vi "Do Local Msg Set.vi"(10 "Variant (X Actor.lvclass)":variant) -> (2 "Local Msg Set":T1)   [LabVIEW 2025, in "jettl.lvlib" / "Actor.lvlib"]
uses:
  Actor.lvlib
  Msg Set.ctl
  Msg/Msg.lvclass
  <vilib>/Utility/Data Type/NI_Data Type.lvlib
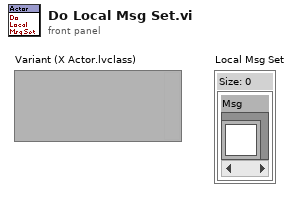
[diagram p1: front panel]
types:
  T1 = typedef "jettl.lvlib/Actor.lvlib/Msg Set.ctl" = set{refnum<class "Msg.lvclass">}
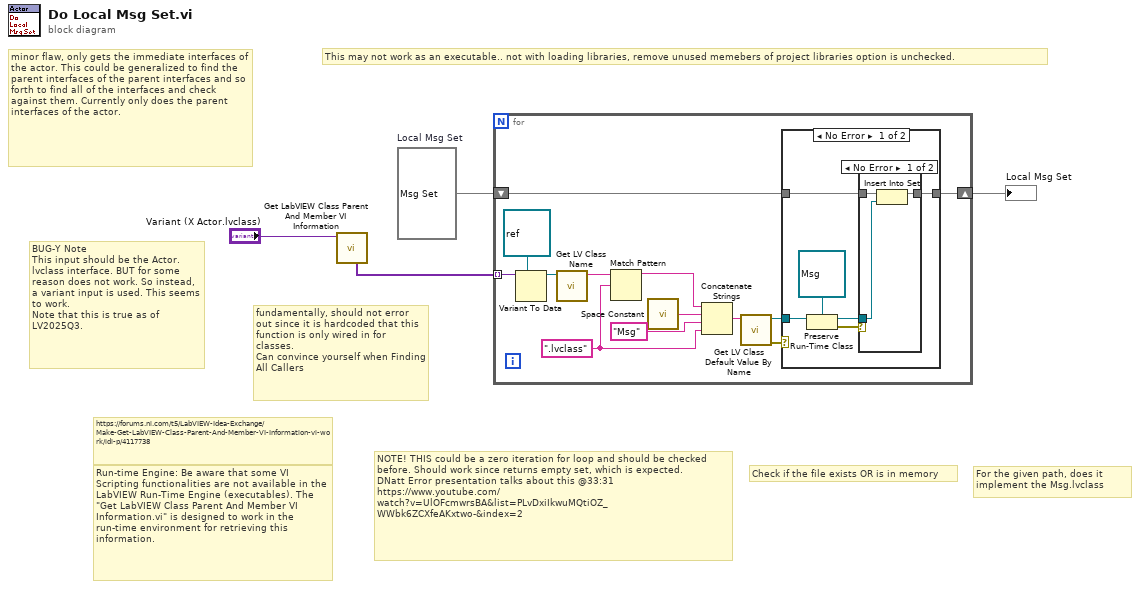
[diagram p0: block diagram]
diagram:
  w1 = T1 {}  # Local Msg Set
  # "fundamentally, should not error out since it is hardcoded that this function is only wired in for classes.\nCan convince yourself when Finding All Callers"
  # "Check if the file exists OR is in memory"
  # "For the given path, does it implement the Msg.lvclass"
  # "NOTE! THIS could be a zero iteration for loop and should be checked before. Should work since returns empty set, which is expected.\nDNatt Error presentation talks about this @33:31\nhttps://www.youtube.com/watch?v=UlOFcmwrsBA&list=PLvDxiIkwuMQtiOZ_WWbk6ZCXfeAKxtwo-&index=2"
  # "BUG-Y Note\nThis input should be the Actor.lvclass interface. BUT for some reason does not work. So instead, a variant input is used. This seems to work.\nNote that this is true as of LV2025Q3."
  # "minor flaw, only gets the immediate interfaces of the actor. This could be generalized to find the parent interfaces of the parent interfaces and so forth to find all of the interfaces and check against them. Currently only does the parent interfaces of the actor."
  # "This may not work as an executable.. not with loading libraries, remove unused memebers of project libraries option is unchecked."
  # "Run-time Engine: Be aware that some VI Scripting functionalities are not available in the LabVIEW Run-Time Engine (executables). The \"Get LabVIEW Class Parent And Member VI Information.vi\" is designed to work in the run-time environment for retrieving this information."
  # "https://forums.ni.com/t5/LabVIEW-Idea-Exchange/Make-Get-LabVIEW-Class-Parent-And-Member-VI-Information-vi-work/idi-p/4117738"
  n1 = call <vilib>:"Get LabVIEW Class Parent And Member VI Information.vi"("variant"="Variant (X Actor.lvclass)") -> ("parent interfaces"=w4:variant[])  [unwired: 7 in, 3 out]
  n2 = for {
    tunnel: w4 -> [w16] mode=indexing
    shift-right: [w12] -> w3
    shift-left: w1 -> [w13]
    w9 = ".lvclass" ("string")
    n3 = Variant To Data(type=refnum<class> refnum ("LabVIEW Object"), Variant=w16) -> (data=w15:refnum<class>)  [unwired: 1 in, 1 out]
    n4 = call <vilib>:"Get LV Class Name.vi"("object"=w15) -> ("class name"=w11:string)  [unwired: 9 in, 1 out]
    n5 = Match Pattern(string=w11, regular expression=w9) -> (before substring=w8:string)  [unwired: 1 in, 3 out]
    n6 = call <vilib>:"Space Constant.vi"() -> ("String"=w7:string)
    n7 = Concatenate Strings(w8, w7, "Msg" ("string"), w9) -> (w6:string)
    n8 = call <vilib>:"Get LV Class Default Value By Name.vi"("class name"=w6) -> ("error out"=w5:errorcluster, "object"=w14:refnum<class>)  [unwired: 9 in]
    n9 = case shown="No Error" w5 {
      tunnel: w14 -> [w20 _]
      tunnel: w13 -> [w19 w28]
      tunnel: [w18 w28] -> w12
      frame No Error {
        n10 = Preserve Run-Time Class(object in=w20, 2:refnum<class "Msg.lvclass"> refnum ("Msg")) -> (object out=w23:refnum<class "Msg.lvclass">, error out=w21:errorcluster)  [unwired: 1 in]
        n11 = case shown="No Error" w21 {
          tunnel: w19 -> [w26 w27]
          tunnel: [w25 w27] -> w18
          tunnel: w23 -> [w24 _]
          frame No Error {
            n12 = Insert Into Set(10:w24, 11:w26) -> (3:w25:T1)  [unwired: 1 out]
          }
          frame Error {
          }
        }
      }
      frame Error {
      }
    }
  }
  "Local Msg Set" <- w3
